vi "print metal-MultiPulses.vi"() -> ()   [LabVIEW 2020]
panel:
  in  "Pulse sepration（毫秒）":u32
  in  "Number of pulses":i32
  in  "Pulse width（毫秒）":u32
  in  "Pulse Voltage(V)":dbl
  in  "Trigger":bool
  in  "退出程序":bool
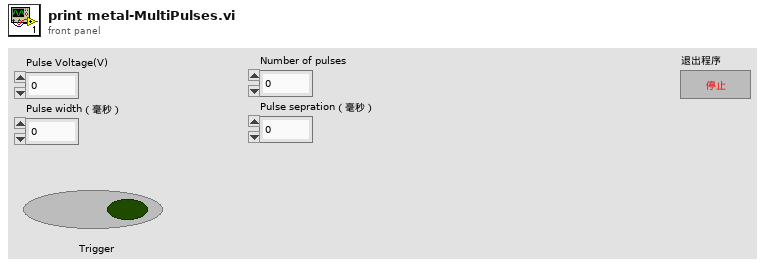
[diagram p1: front panel]
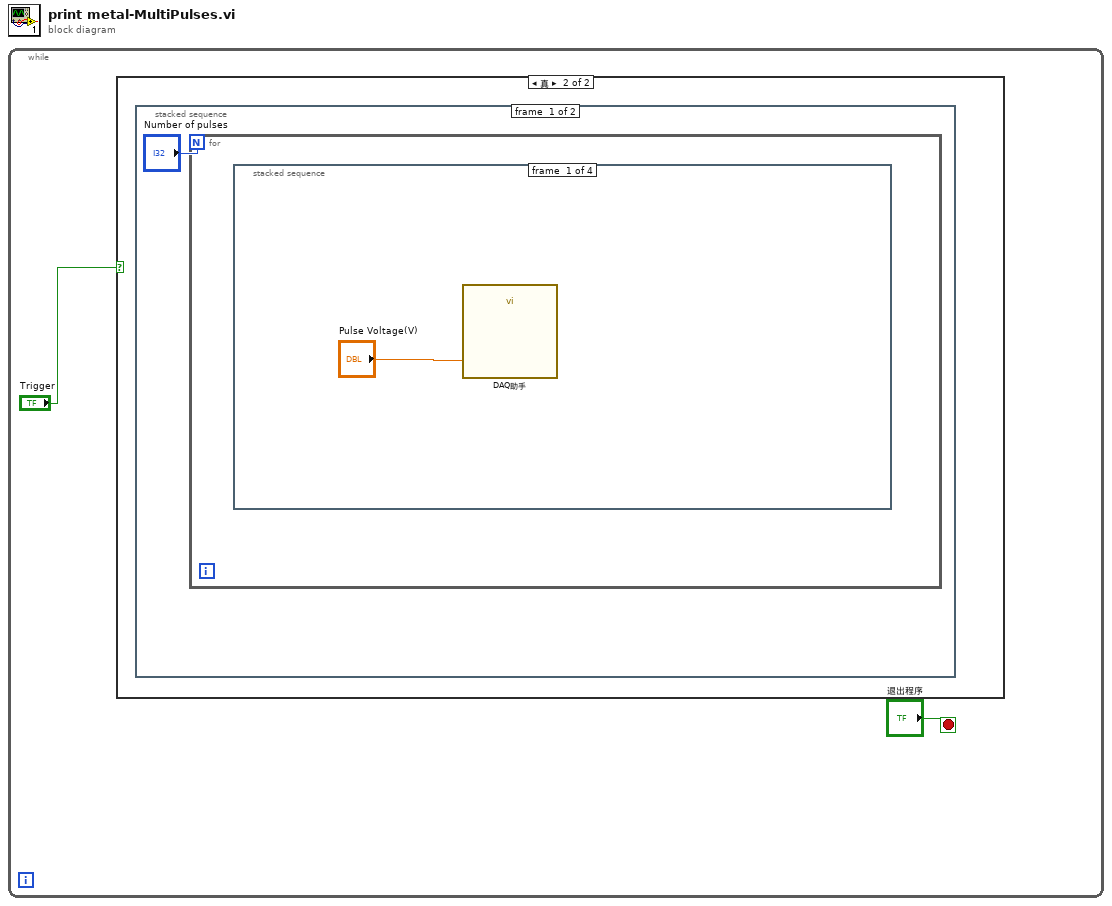
[diagram p0: block diagram]
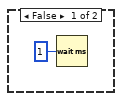
[diagram p2: hidden frame]
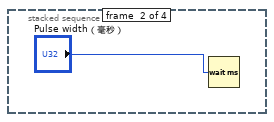
[diagram p3: hidden frame]
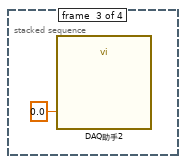
[diagram p4: hidden frame]
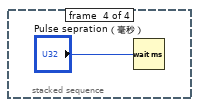
[diagram p5: hidden frame]
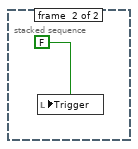
[diagram p6: hidden frame]
diagram:
  n1 = while {
    stop <- "退出程序" stop-if-true
    n2 = case shown="真" "Trigger" {
      frame False {
        n3 = Wait (ms)(milliseconds to wait=u32 1 ("等待时间（毫秒）")) -> ()  [unwired: 1 out]
      }
      frame True {
        n4 = stacked-sequence {
          frame #0 {
            n5 = for {
              N: "Number of pulses" -> [_]
              n6 = stacked-sequence {
                frame #0 {
                  n7 = call "DAQ助手"("data"="Pulse Voltage(V)") -> ()  [unwired: 17 in, 2 out]
                }
                frame #1 {
                  n8 = Wait (ms)(milliseconds to wait="Pulse width（毫秒）") -> ()  [unwired: 1 out]
                }
                frame #2 {
                  n9 = call "DAQ助手2"("data"=0.0) -> ()  [unwired: 17 in, 2 out]
                }
                frame #3 {
                  n10 = Wait (ms)(milliseconds to wait="Pulse sepration（毫秒）") -> ()  [unwired: 1 out]
                }
              }
            }
          }
          frame #1 {
            n11 = local write "Trigger"(FALSE) -> ()
          }
        }
      }
    }
  }
